vi "Start Default Sync.vi"(8 "error in (no error)":errorcluster, 11 "gRPC Server in":refnum<class "Data Marshal Server.lvclass">) -> (0 "error out":errorcluster, 3 "gRPC Server out":refnum<class "Data Marshal Server.lvclass">)   [LabVIEW 2019, in "Data Marshal Server.lvlib" / "Data Marshal Server.lvclass"]
uses:
  Data Marshal Server.lvclass
  Data Marshal Server.lvclass/Data Marshal Server.ctl
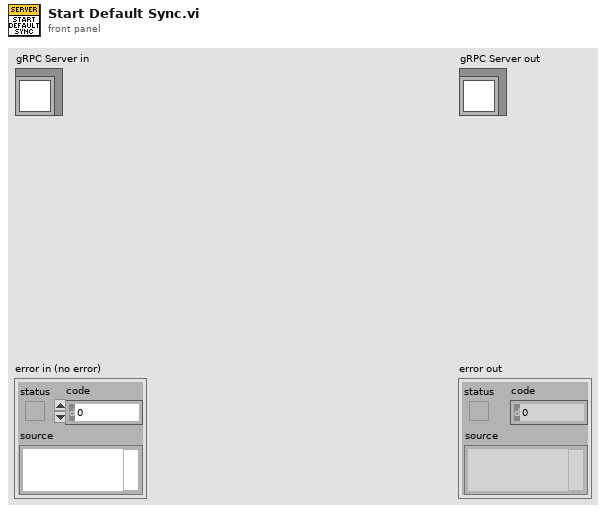
[diagram p1: front panel]
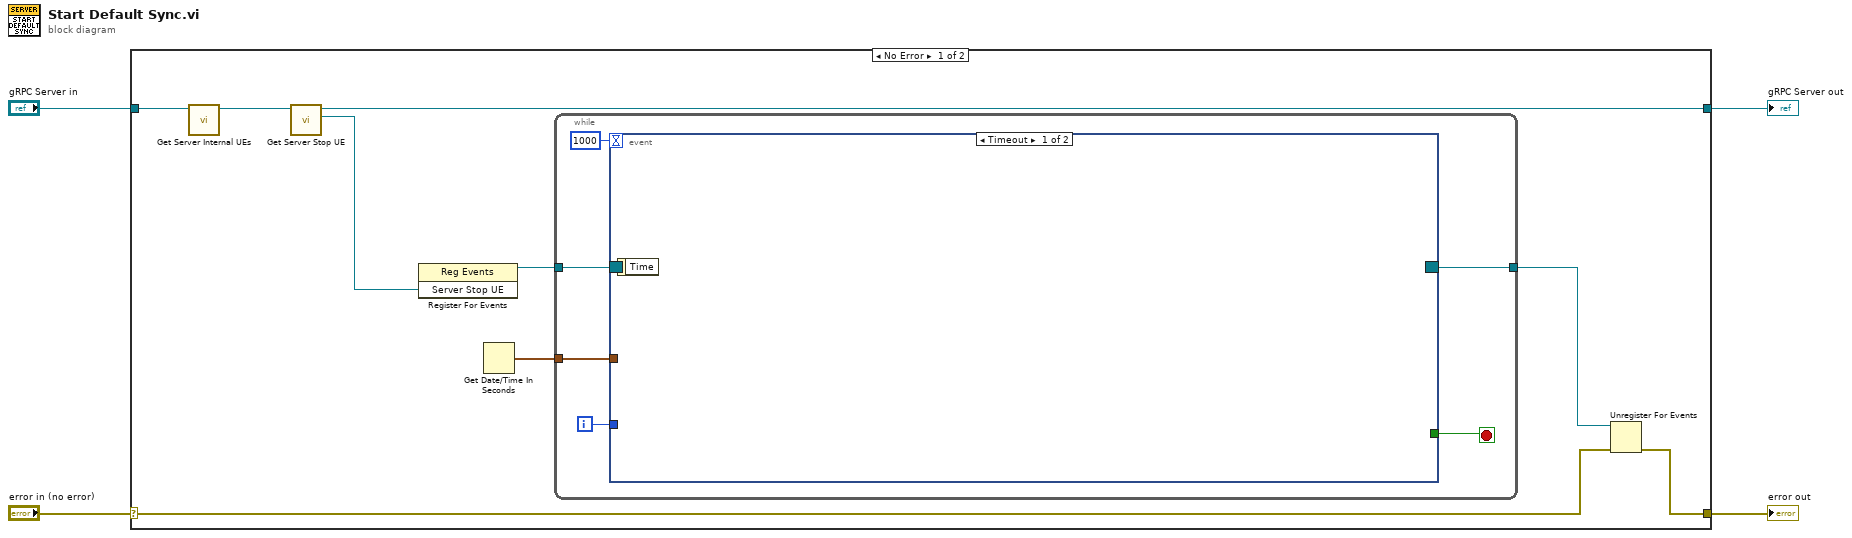
[diagram p0: block diagram]
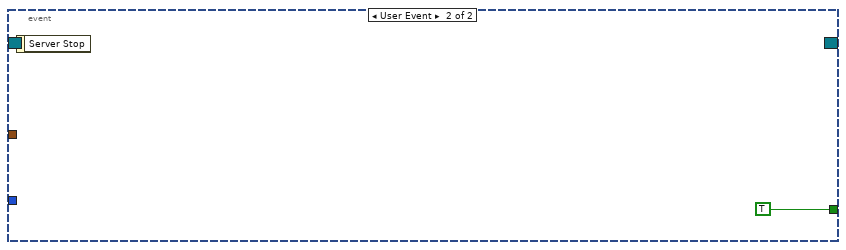
[diagram p2: hidden frame]
diagram:
  n1 = case shown="No Error" "error in (no error)" {
    selector: "error in (no error)" -> [w9 w22]
    tunnel: [w8 w22] -> w3
    tunnel: [w12 w21] -> w1
    tunnel: "gRPC Server in" -> [w6 w21]
    frame No Error {
      n2 = call "Get Server Internal UEs.vi"("OOP Server in"=w6) -> ("OOP Server out"=w5:refnum<class "Data Marshal Server.lvclass">)  [unwired: 9 in, 1 out]
      n3 = call "Get Server Stop UE.vi"("OOP Server in"=w5) -> ("Server Stop UE"=w13:refnum<user-event>, "OOP Server out"=w12:refnum<class "Data Marshal Server.lvclass">)  [unwired: 9 in]
      n4 = register-events(w13) -> (reference out=w11:refnum<event-registration>)  [unwired: 2 in, 1 out]
      n5 = Get Date/Time In Seconds() -> (seconds since 1Jan1904=w7:timestamp)
      n6 = while {
        tunnel: w11 -> [w19]
        tunnel: [w17] -> w10
        tunnel: w7 -> [w16]
        i -> [w15]
        stop <- w18 stop-if-true
        n7 = event shown="[0] Timeout" {
          selector: w19 -> [_ _]
          dyn-events: [_ _] -> w17
          timeout: 1000 -> [_ _]
          tunnel: [_ TRUE] -> w18
          tunnel: w16 -> [_ _]
          tunnel: w15 -> [_ _]
          event Timeout {
            n8 = event-data() -> ()  [unwired: 1 in, 1 out]
          }
          event User Event {
            n9 = event-data() -> ()  [unwired: 1 in, 1 out]
          }
        }
      }
      n10 = Unregister For Events(event registration refnum=w10, error in=w9) -> (error out=w8:errorcluster)
    }
    frame Error {
    }
  }
  "error out" <- w3
  "gRPC Server out" <- w1
